vi "Tester - Get LCD Image.vi"(8 "error in (no error)":errorcluster, 11 "VISA resource name":refnum<visa-resource-name>) -> (0 "error out":errorcluster, 2 "24-bit pixmap":u32[][](array[numeric]), 3 "VISA resource name out":refnum<visa-resource-name>)   [LabVIEW 2011]
uses:
  Video Hardware Simulation Commands.ctl
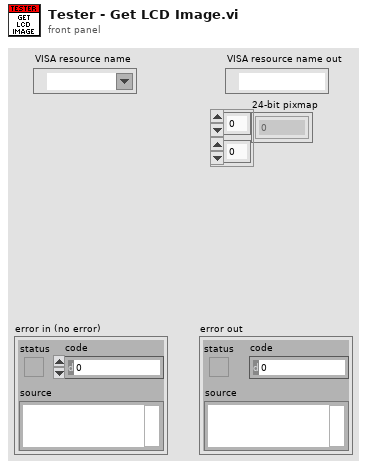
[diagram p1: front panel]
types:
  T1 = typedef "Video Hardware Simulation Commands.ctl" = enum16{"Simulate Generate Video Output", "Simulate Read HDMI Data"}
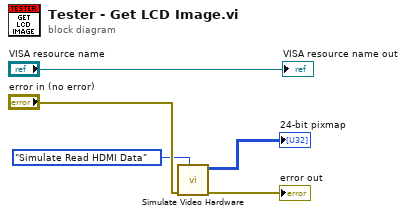
[diagram p0: block diagram]
diagram:
  n1 = call "Simulate Video Hardware.vi"("Command to Simulate"=Video_Hardware_Simulation_Commands."Simulate Read HDMI Data", "error in (no error)"="error in (no error)") -> ("error out"=→"error out":errorcluster, "UUT Image Data Out"=→"24-bit pixmap":u32[][])  [unwired: 8 in]
  "VISA resource name out" <- "VISA resource name"
